vi "RFSG CW Generation.vi"(11 "Frequency (Hz)":dbl=1000000000.0 format="%#.3p") -> (0 "error out":errorcluster {"code" format="%.0x"})   [LabVIEW 2019]
doc: "Demonstrates how to generate a single tone CW at a specified frequency and power."
uses:
  <instrlib>/niRFSG/niRFSG.llb/niRFSG Ref Clock Sources.ctl
panel:
  in  "Clock Source":T1="OnboardClock"
  in  "Resource Name":refnum<k15>="5652" caption="resource name"
  in  "Power Level (dBm)":dbl=-5.0 format="%_3f"
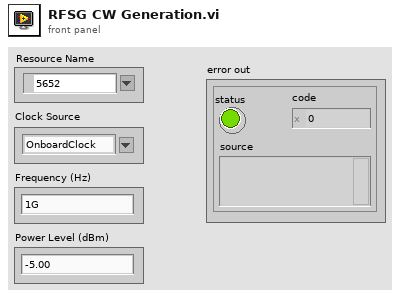
[diagram p1: front panel]
types:
  T1 = typedef "niRFSG Ref Clock Sources.ctl" = string
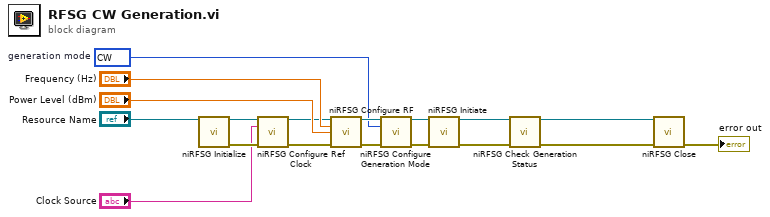
[diagram p0: block diagram]
diagram:
  w11 = 1000 items=["CW"=1000, "Arb Waveform"=1001, "Script"=1002]  # generation mode
  n1 = call <instrlib>:"niRFSG Initialize.vi"("resource name"="Resource Name") -> ("instrument handle"=w18:refnum<k15>, "error out"=w6:errorcluster)  [unwired: 13 in]
  n2 = call <instrlib>:"niRFSG Configure Ref Clock.vi"("instrument handle"=w18, "ref clock source"="Clock Source", "error in"=w6) -> ("instrument handle out"=w7:refnum<k15>, "error out"=w5:errorcluster)  [unwired: 11 in]
  n3 = call <instrlib>:"niRFSG Configure RF.vi"("instrument handle"=w7, "frequency (Hz)"="Frequency (Hz)", "power level (dBm)"="Power Level (dBm)", "error in"=w5) -> ("instrument handle out"=w12:refnum<k15>, "error out"=w15:errorcluster)  [unwired: 10 in]
  n4 = call <instrlib>:"niRFSG Configure Generation Mode.vi"("instrument handle"=w12, "generation mode"=w11, "error in"=w15) -> ("instrument handle out"=w13:refnum<k15>, "error out"=w14:errorcluster)  [unwired: 11 in]
  n5 = call <instrlib>:"niRFSG Initiate.vi"("instrument handle"=w13, "error in"=w14) -> ("instrument handle out"=w17:refnum<k15>, "error out"=w2:errorcluster)  [unwired: 12 in]
  n6 = call <instrlib>:"niRFSG Check Generation Status.vi"("instrument handle"=w17, "error in"=w2) -> ("instrument handle out"=w16:refnum<k15>, "error out"=w3:errorcluster)  [unwired: 11 in, 1 out]
  n7 = call <instrlib>:"niRFSG Close.vi"("instrument handle"=w16, "error in"=w3) -> ("error out"=→"error out":errorcluster)  [unwired: 13 in]
